vi "TranslatorBooster Build VI Inputs and Outputs.vi"(8 "error in (no error)":errorcluster, 10 "Function parameters":string[](array[string]), 11 "VI in":refnum<vi>) -> (0 "error out":errorcluster, 3 "VI out":refnum<vi>)   [LabVIEW 2014, in "Complex Numbers.lvlib"]
uses:
  <vilib>/Aledyne-TSXperts/Arduino Compatible Compiler for LabVIEW/addons/Complex Numbers/Complex Numbers.lvlib
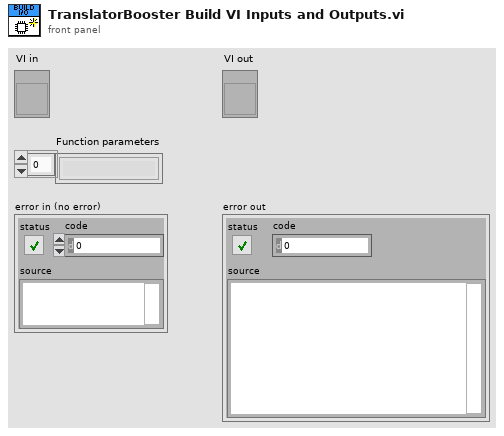
[diagram p1: front panel]
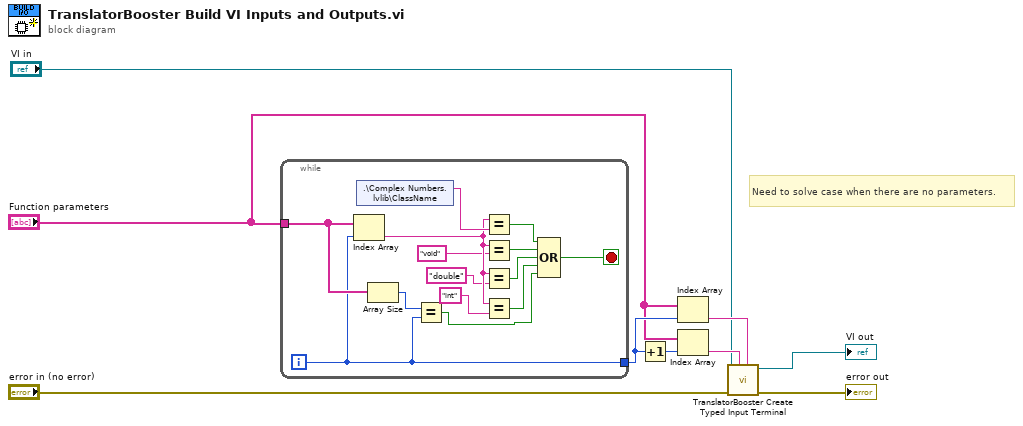
[diagram p0: block diagram]
diagram:
  # "Need to solve case when there are no parameters."
  n1 = while {
    tunnel: "Function parameters" -> [w23]
    tunnel: [w10] -> w5
    i -> [w10]
    stop <- w11 stop-if-true
    n2 = Index Array(array=w23, index=w10) -> (element=w20:string)
    n3 = shared-variable ".\\Complex Numbers.lvlib\\ClassName"() -> (w21:string)  [unwired: 1 in, 1 out]
    n4 = Array Size(array=w23) -> (size(s)=w22:i32)
    n5 = Equal?(x=w22, y=w10) -> (x = y?=w12:bool)
    n6 = Equal?(x=w20, y=w21) -> (x = y?=w16:bool)
    n7 = Equal?(x=w20, y="void") -> (x = y?=w15:bool)
    n8 = Equal?(x=w20, y="double") -> (x = y?=w14:bool)
    n9 = Equal?(x=w20, y="int") -> (x = y?=w13:bool)
    n10 = Compound Arithmetic op=OR(w16, w15, w14, w13, w12) -> (w11:bool)
  }
  n11 = Increment(x=w5) -> (x+1=w4:i32)
  n12 = Index Array(array="Function parameters", index=w5) -> (element=w7:string)
  n13 = Index Array(array="Function parameters", index=w4) -> (element=w6:string)
  n14 = call <vilib>:"TranslatorBooster Create Typed Input Terminal.vi"("Param type"=w7, "Input name"=w6, "Error In"="error in (no error)", "parent VI"="VI in") -> ("Error Out"=→"error out":errorcluster, "parent VI out"=→"VI out":refnum<vi>)  [unwired: 6 in]
